vi "Extract Double From String.vi"(0 "string":string, 1 "start index":i32) -> (2 "valid":bool, 3 "floating pt. number":dbl format="%.2f", 4 "end index":i32)   [LabVIEW 2016]
doc: "Scan any string for a number, beginning at the input index. Any of the following formats are recognized:\n123 1.23 1.23e2 1.23E2\nNo spaces or other characters may appear within the number, but any characters may appear before or after the number. Returns true if a number is found, the value of the number, and the index of the first character after the number."
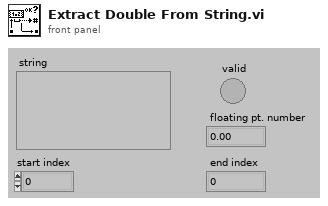
[diagram p1: front panel]
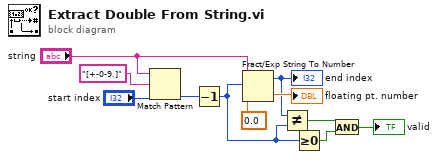
[diagram p0: block diagram]
diagram:
  n1 = Match Pattern(string="string", regular expression="[+-0-9.]", offset (0)="start index") -> (offset past match=w10:i32)  [unwired: 3 out]
  n2 = Decrement(x=w10) -> (x-1=w5:i32)
  n3 = Fract/Exp String To Number(string="string", offset=w5, default (0 dbl)=0.0) -> (offset past number=w4:i32, number=→"floating pt. number":dbl)  [unwired: 1 in]
  "end index" <- w4
  n4 = Not Equal?(x=w4, y=w5) -> (x != y?=w3:bool)
  n5 = Greater Or Equal To 0?(x=w5) -> (x >= 0?=w2:bool)
  n6 = And(x=w3, y=w2) -> (x .and. y?=→"valid":bool)
